vi "WriteMotorState.vi"(8 "error in (no error)":errorcluster, 10 "MCSA FFT":T1[](array[typedef]), 11 "map in":T2) -> (0 "error out":errorcluster, 3 "map out":T2)   [LabVIEW 2017, in "McsaAnalysisFunctions.lvlib"]
uses:
  <vilib>/addons/InsightCM/Utilities/Analysis/MCSA/McsaAnalysisFunctions.lvlib
  <vilib>/addons/PointValueMap/controls/PointMap.ctl
  <vilib>/addons/InsightCM/Utilities/Analysis/MCSA/controls/MotorState.ctl
  <vilib>/addons/PointValueMap/subVIs/Point_Write_variant.vi
  <vilib>/addons/PointValueMap/PointValueMap.lvlib
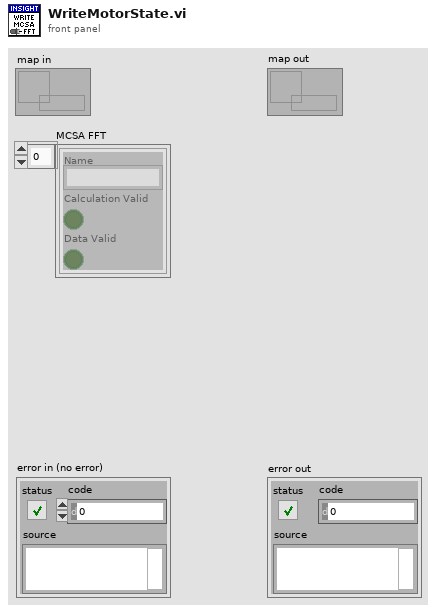
[diagram p1: front panel]
types:
  T1 = typedef "McsaAnalysisFunctions.lvlib/MotorState.ctl" = cluster{"Name":string, "Calculation Valid":bool, "Data Valid":bool}
  T2 = typedef "PointValueMap.lvlib/PointMap.ctl" = refnum<data-value>
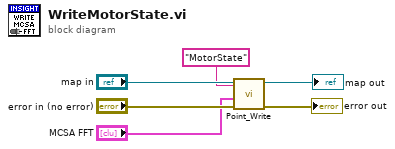
[diagram p0: block diagram]
diagram:
  n1 = call-poly <vilib>:"Point_Write.vi"("Error In"="error in (no error)", "Value"="MCSA FFT", "Tag"="MotorState", "Map"="map in") -> ("Error Out"=→"error out":errorcluster, "Map Out"=→"map out":T2)  [unwired: 6 in]
